vi "cleanTCPQueue.vi"(8 "error in (no error)":errorcluster, 11 "SpectrographClientCommunicator in":refnum<class "SpectrographClientCommunicator.lvclass">) -> (0 "error out":errorcluster, 2 "message":string, 3 "SpectrographClientCommunicator out":refnum<class "SpectrographClientCommunicator.lvclass">)   [LabVIEW 2016, in "SpectrographClientCommunicator.lvclass"]
uses:
  SpectrographClientCommunicator.lvclass
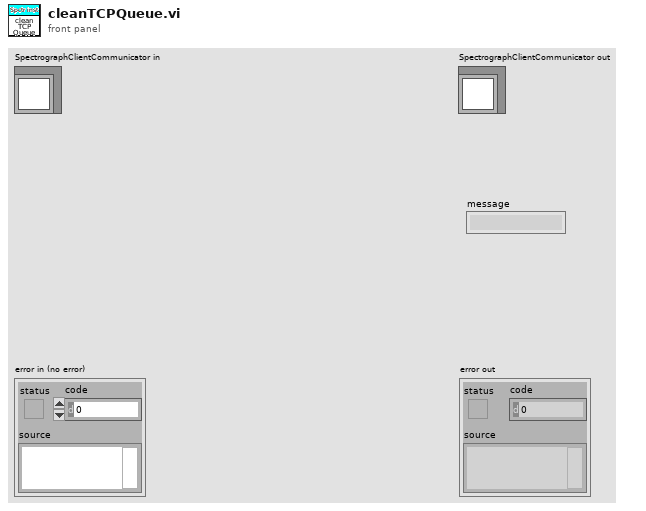
[diagram p1: front panel]
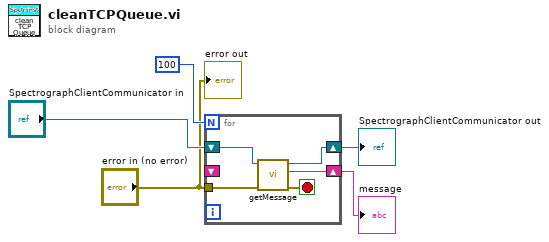
[diagram p0: block diagram]
diagram:
  n1 = for {
    N: 100 -> [_]
    tunnel: "error in (no error)" -> [w9]
    shift-right: [w7] -> w2
    shift-left: "SpectrographClientCommunicator in" -> [w8]
    shift-right: [w6] -> w1
    shift-left: _ -> [_]
    stop <- w10 stop-if-true
    n2 = call "getMessage.vi"("error in (no error)"=w9, "SpectrographClientCommunicator in"=w8) -> ("error out"=w10:errorcluster, "message"=w6:string, "SpectrographClientCommunicator out"=w7:refnum<class "SpectrographClientCommunicator.lvclass">)  [unwired: 7 in]
  }
  "SpectrographClientCommunicator out" <- w2
  "message" <- w1
  "error out" <- "error in (no error)"
